vi "Nano-drive.vi"(0 "X (um)":ext format="%.4f", 2 "Y (um)":ext format="%.4f", 3 "Z (um)":ext format="%.4f", 4 "Set this axis?":cluster{"X":bool, "Y":bool, "Z":bool}) -> ()   [LabVIEW 2011]
doc: "Moves the Mad City piezo stage by a fixed amount in x, y, and z"
uses:
  new-h-nu-ixon/stage globals.vi
  Program Files (x86)/Gelles Lab Software/Madlib.dll
panel:
  out "z readout":dbl
  out "y readout":dbl
  out "x readout":dbl
  # "Specific for Mad City USB controller"
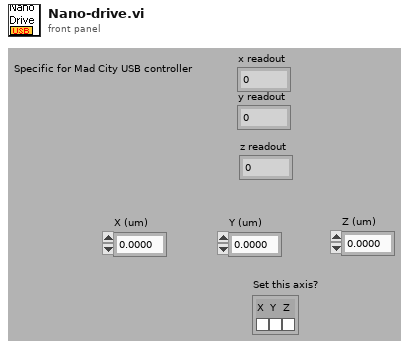
[diagram p1: front panel]
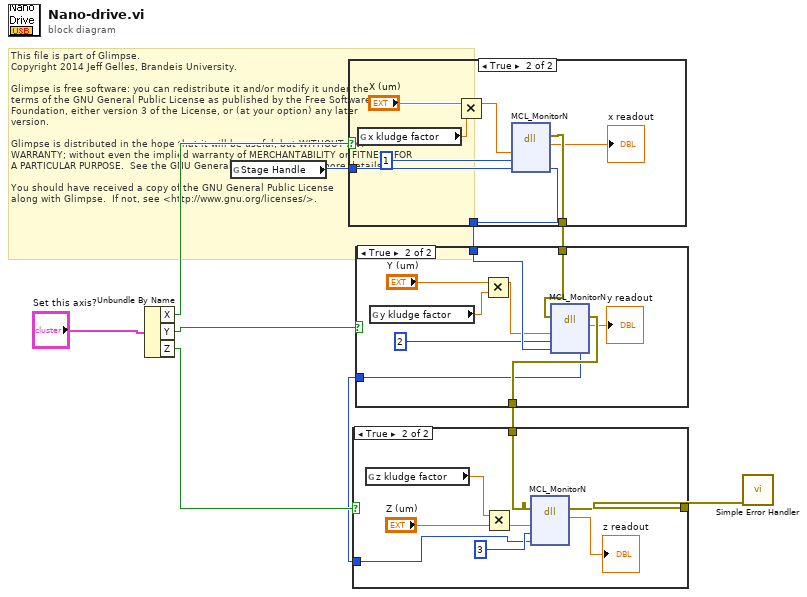
[diagram p0: block diagram]
diagram:
  # "This file is part of Glimpse. \nCopyright 2014 Jeff Gelles, Brandeis University.    \n\nGlimpse is free software: you can redistribute it and/or modify it under the \nterms of the GNU General Public License as published by the Free Software \nFoundation, either version 3 of the License, or (at your option) any later \nversion.\n\nGlimpse is distributed in the hope that it will be useful, but WITHOUT ANY \nWARRANTY; without even the implied warranty of MERCHANTABILITY or FITNESS FOR \nA PARTICULAR PURPOSE.  See the GNU General Public License for more details.\n\nYou should have received a copy of the GNU General Public License\nalong with Glimpse.  If not, see <http://www.gnu.org/licenses/>."
  n1 = Unbundle By Name("Set this axis?") -> ("X"=w9:bool, "Y"=w8:bool, "Z"=w7:bool)
  n2 = global read "stage globals.vi" "Stage Handle"() -> (w3:i32)
  n3 = case shown="True" w9 {
    tunnel: [_ w19] -> w6
    tunnel: w3 -> [w11 w16]
    tunnel: [w11 w15] -> w2
    frame False {
    }
    frame True {
      n4 = global read "stage globals.vi" "x kludge factor"() -> (w12:ext)
      n5 = Multiply(x="X (um)", y=w12) -> (x*y=w13:ext)
      n6 = dll-call lib="C:/Program Files (x86)/Gelles Lab Software/MADLib.dll" fn="MCL_MonitorN"("position"=w13, "axis"=1, "handle"=w16) -> (error out=w19:errorcluster, "return type"=→"x readout":dbl, "handle"=w15:i32)  [unwired: 5 in, 1 out]
    }
  }
  n7 = case shown="True" w8 {
    tunnel: w6 -> [w21 w30]
    tunnel: [w21 w29] -> w5
    tunnel: w2 -> [w20 w27]
    tunnel: [w20 w25] -> w1
    frame False {
    }
    frame True {
      n8 = global read "stage globals.vi" "y kludge factor"() -> (w22:ext)
      n9 = Multiply(x="Y (um)", y=w22) -> (x*y=w23:ext)
      n10 = dll-call lib="C:/Program Files (x86)/Gelles Lab Software/MADLib.dll" fn="MCL_MonitorN"(error in=w30, "position"=w23, "axis"=2, "handle"=w27) -> (error out=w29:errorcluster, "return type"=→"y readout":dbl, "handle"=w25:i32)  [unwired: 4 in, 1 out]
    }
  }
  n11 = case shown="True" w7 {
    tunnel: w5 -> [w31 w38]
    tunnel: [w31 w39] -> w4
    tunnel: w1 -> [_ w35]
    frame False {
    }
    frame True {
      n12 = global read "stage globals.vi" "z kludge factor"() -> (w32:ext)
      n13 = Multiply(x=w32, y="Z (um)") -> (x*y=w33:ext)
      n14 = dll-call lib="C:/Program Files (x86)/Gelles Lab Software/MADLib.dll" fn="MCL_MonitorN"(error in=w38, "position"=w33, "axis"=3, "handle"=w35) -> (error out=w39:errorcluster, "return type"=→"z readout":dbl)  [unwired: 5 in, 1 out]
    }
  }
  n15 = call <vilib>:"Simple Error Handler.vi"("error in (no error)"=w4) -> ()  [unwired: 1 in, 8 out]
